vi "Power.vi"(5 "Negative Power":dbl, 7 "Positive Power":dbl, 9 "Negative":bool, 10 "Positive":bool) -> (2 "Output":dbl)   [LabVIEW 2018]
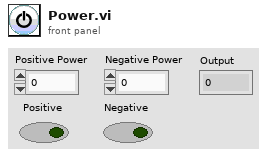
[diagram p1: front panel]
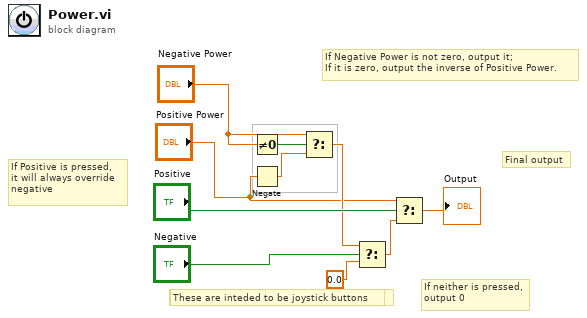
[diagram p0: block diagram]
diagram:
  # "These are intended to be joystick buttons."
  # "Final output"
  # "If neither is pressed,\noutput 0"
  # "If Positive is pressed, \nit will always override \nnegative"
  # "If Negative Power is not zero, output it;\nIf it is zero, output the inverse of Positive Power."
  # "These are inteded to be joystick buttons"
  n1 = Not Equal To 0?(x="Negative Power") -> (x != 0?=w5:bool)
  n2 = Negate(x="Positive Power") -> (-x=w2:dbl)
  n3 = Select(t="Negative Power", s=w5, f=w2) -> (s? t:f=w3:dbl)
  n4 = Select(t=w3, s="Negative", f=0.0) -> (s? t:f=w10:dbl)
  n5 = Select(t="Positive Power", s="Positive", f=w10) -> (s? t:f=→"Output":dbl)
